vi "Actor Core.vi"(8 "error in":errorcluster, 11 "LabActor in":refnum<class "LabActor.lvclass">) -> (0 "error out":errorcluster, 3 "Actor out":refnum<class "Actor.lvclass">)   [LabVIEW 2020, in "LabActor.lvclass"]
doc: "(<B>Filename</B>: Actor Framework.lvlib:Actor.lvclass:Actor Core.vi)\n\nReceives messages to the actor, reacts to them, and initiates any error handling that may shut the actor down.\n\nDescendant classes may override this VI to append parallel tasks for the actor to complete while it handles messages. Overrides use the Call Parent Method node."
uses:
  LabActor.lvclass
  C:/GitHub/LabActor/Controllers/Application Controller/Application Controller.lvclass
  C:/GitHub/LabActor/Template Module/Template Module.lvclass
  C:/Program Files/National Instruments/LabVIEW 2020/vi.lib/ActorFramework/Actor/Actor.lvclass
  <vilib>/ActorFramework/Actor/Actor.lvclass
  NHMFL_Core/Libraries/Queued Listbox/Queued Listbox.xctl
  <vilib>/Utility/miscctls.llb/LVRectTypeDef.ctl
  <vilib>/Utility/miscctls.llb/LVPointTypeDef.ctl
  LabActor.lvclass/LabActor.ctl
  Controllers/Application Controller/Application Controller.lvclass/Application Controller.ctl
  Template Module/Template Module.lvclass/Template Module.ctl
  <vilib>/ActorFramework/Actor/Actor.lvclass/Actor.ctl
  <vilib>/ActorFramework/Message Enqueuer/Message Enqueuer.lvclass/Message Enqueuer.ctl
  Controllers/Application Controller Messages/Pulse Acquired Result/Pulse Acquired Result.lvclass
  C:/GitHub/LabActor/Template Module Messages/Result Reply Msg/Result Reply Msg.lvclass
  Controllers/Application Controller Messages/Pulse Acquired Result/Pulse Acquired Result.lvclass/Pulse Acquired Result.ctl
  LabActor Messages/Start Pulse Measurements Msg/Start Measurements Command Msg.lvclass/Start Measurements Command Msg.ctl
  LabActor Messages/Stop Measurements Command Msg/Stop Measurements Command Msg.lvclass/Stop Measurements Command Msg.ctl
  Worker Messages/Pause Work Msg/Pause Work Msg.lvclass
  C:/Program Files/National Instruments/LabVIEW 2020/vi.lib/ActorFramework/Message/Message.lvclass
  Worker Messages/Un-Pause Work Msg/Un-Pause Work Msg.lvclass
  Template Module Messages/Message Nested Object Msg/Message Nested Object Msg.lvclass/Message Nested Object Msg.ctl
  Template Module Messages/Open Item Msg/Open Item Msg.lvclass/Open Item Msg.ctl
  Template Module Messages/Save Configuration Msg/Save Configuration Msg.lvclass/Save Configuration Msg.ctl
  Plots/Plot types.ctl
  Controllers/Application Controller Messages/Open Waveform File Plot Msg/Open Waveform File Plot Msg.lvclass/Open Waveform File Plot Msg.ctl
  Controllers/Application Controller Messages/Pulse Acquired Result/Write Open plot.vi
  Controllers/Application Controller/Write Armed ref.vi
  Controllers/Application Controller/Write Devices armed.vi
  Controllers/Application Controller/Write Monitor Running.vi
  Controllers/Application Controller/Write Monitor ref.vi
  Controllers/Application Controller/Write Postproc ref.vi
  Template Module/Read stop event.vi
  Template Module/Read Open item event.vi
  Controllers/Application Controller/Read Monitor start event.vi
  Controllers/Application Controller/Read Monitor stop event.vi
  <vilib>/ActorFramework/Message Enqueuer/Init from Existing Queue.vi
  <vilib>/ActorFramework/Message Enqueuer/Enqueue.vi
  <vilib>/ActorFramework/Stop Msg/Stop Msg.lvclass
  LabActor Messages/Start Pulse Measurements Msg/Start Measurements Command Msg.lvclass
  LabActor Messages/Stop Measurements Command Msg/Stop Measurements Command Msg.lvclass
  Template Module Messages/Message Nested Object Msg/Message Nested Object Msg.lvclass
  Template Module Messages/Open Item Msg/Open Item Msg.lvclass
  Template Module Messages/Save Configuration Msg/Save Configuration Msg.lvclass
  Controllers/Application Controller Messages/Open Waveform File Plot Msg/Open Waveform File Plot Msg.lvclass
  <vilib>/ActorFramework/Message Priority Queue/Priority Enqueue.vi
  Controllers/Application Controller/Application Controller.lvclass
  <vilib>/ActorFramework/Message Enqueuer/Message Enqueuer.lvclass
  Template Module Messages/Restore Configuration Msg/Restore Configuration Msg.lvclass
  C:/GitHub/LabActor/Template Module Messages/Self-Addressed Msg/Self-addressed Msg.lvclass
  C:/GitHub/LabActor/Controllers/Application Controller Messages/Pulse Acquired Result/Pulse Acquired Result.lvclass
  C:/GitHub/LabActor/Controllers/Process Controller/Process Controller.lvclass
  C:/GitHub/LabActor/Worker/Worker.lvclass
  C:/GitHub/LabActor/LabActor/LabActor.lvclass
  C:/GitHub/LabActor/Worker Messages/Pause Work Msg/Pause Work Msg.lvclass
  C:/GitHub/LabActor/Worker Messages/Un-Pause Work Msg/Un-Pause Work Msg.lvclass
panel:
  in  "Error log":bool
  out "Origin":T1
  out "Front Panel Window:Panel Bounds":T2
  out "Devices armed":bool[](array[boolean])
  in  "About Button":bool
  in  "Pause":bool
  in  "Disarm":bool
  in  "Full XY Plot":bool
  out "Monitor file":path caption="Monintor\nFile"
  in  "View Waveform":bool
  out "PEAK FIELD":dbl format="%#.2f"
  in  "Exit":bool
  in  "Monitor configuration":bool
  in  "Pulse configuration":bool
  out "Pulse file":path caption="Pulse\nFile"
  in  "Write cfg":bool
  in  "Read cfg":bool
  in  "View XY Plot":bool
  out "Monitor Running":bool
  out "Armed":bool
  in  "Arm":bool
  in  "Stop monitor":bool
  in  "Start monitor":bool
  in  "Monitor":string[](xcontrol)
  in  "Process Pulse":string[](xcontrol)
  in  "Acquire Pulse":string[](xcontrol)
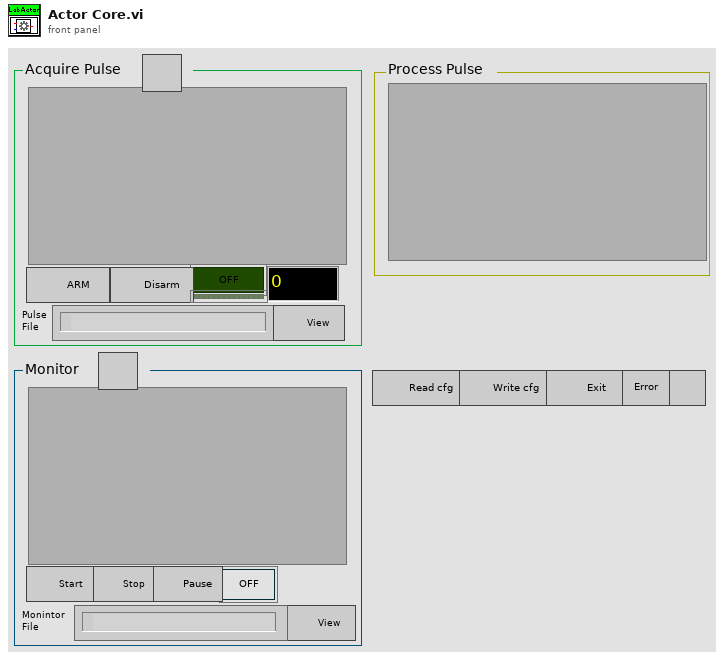
[diagram p1: front panel]
types:
  T1 = typedef "LVPointTypeDef.ctl" = cluster{"Horizontal":i16, "Vertical":i16}
  T2 = typedef "LVRectTypeDef.ctl" = cluster{"Left":i16, "Top":i16, "Right":i16, "Bottom":i16}
  T3 = typedef "Plot types.ctl" = enum16{"Waveform Plot", "XY Plot", "Full XY"}
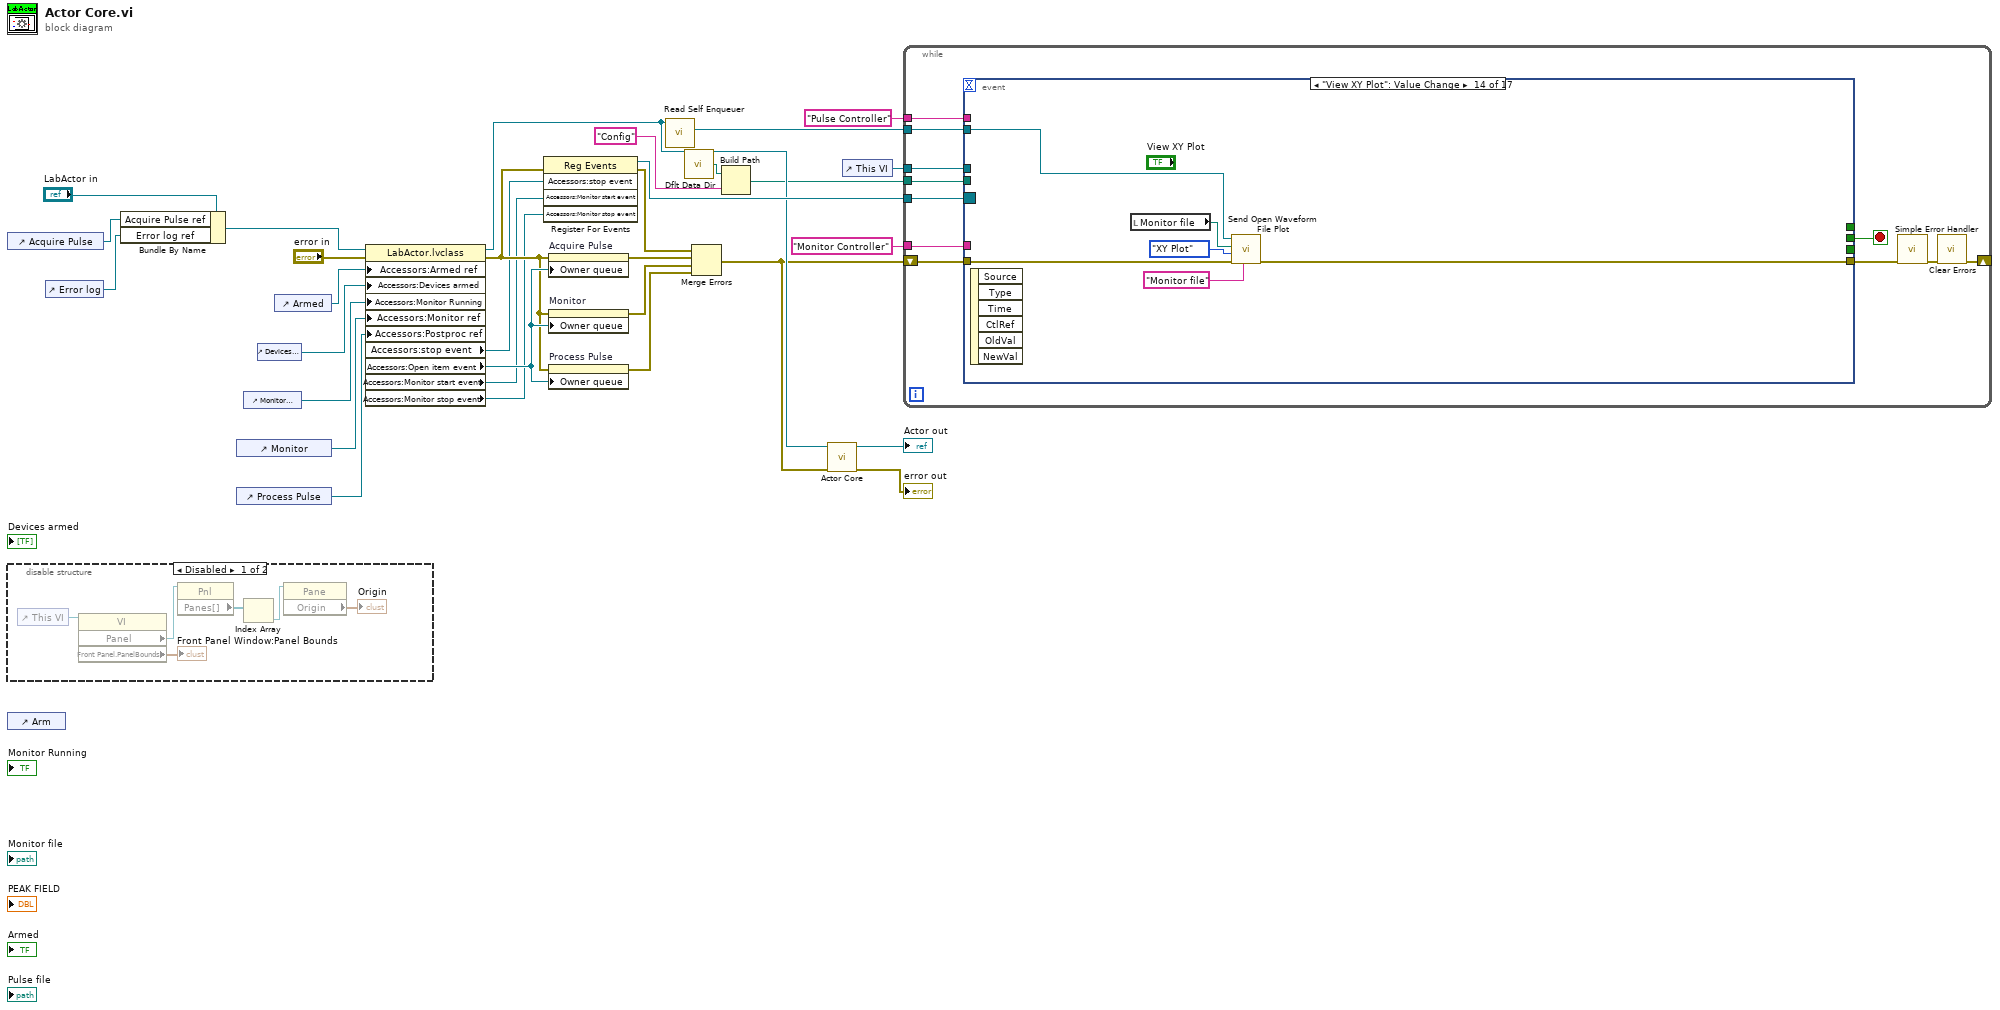
[diagram p0: block diagram]
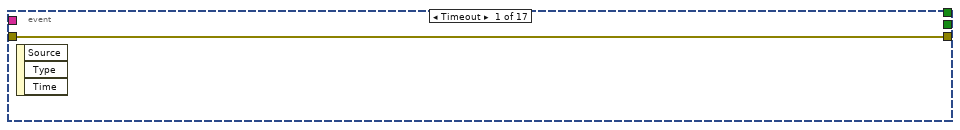
[diagram p3: hidden frame]
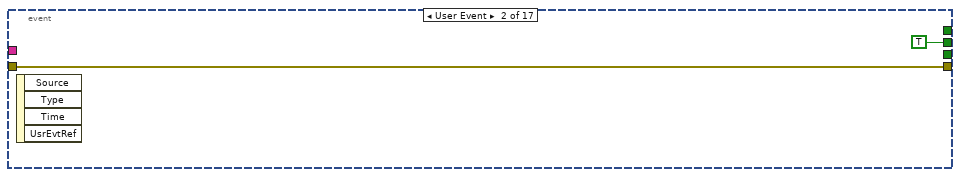
[diagram p4: hidden frame]
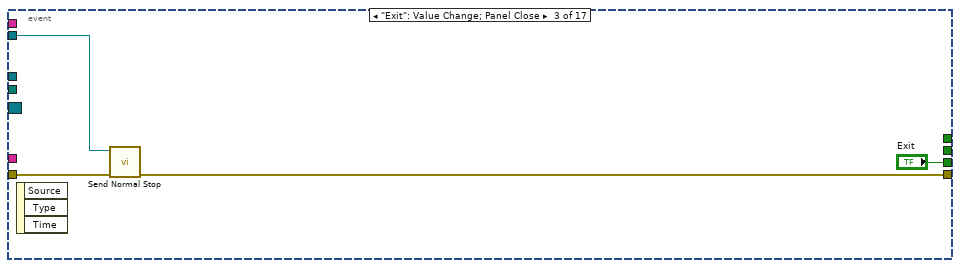
[diagram p5: hidden frame]
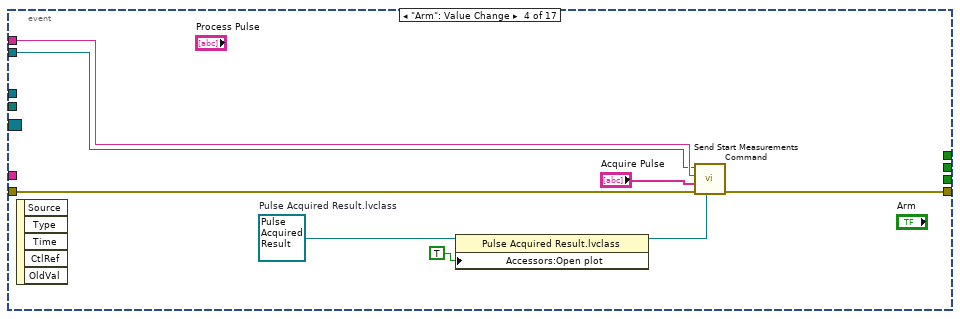
[diagram p6: hidden frame]
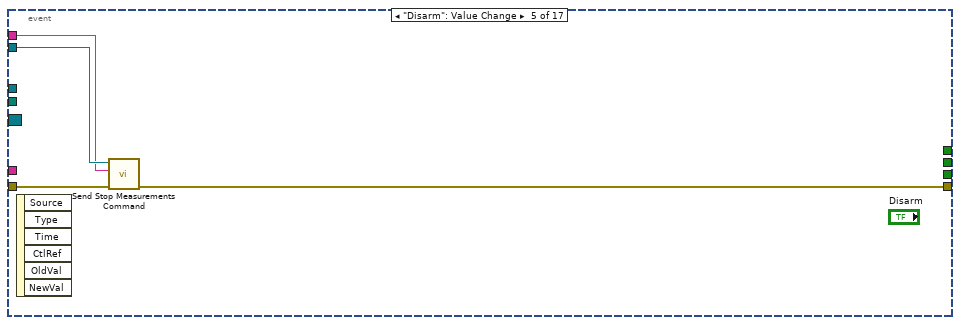
[diagram p7: hidden frame]
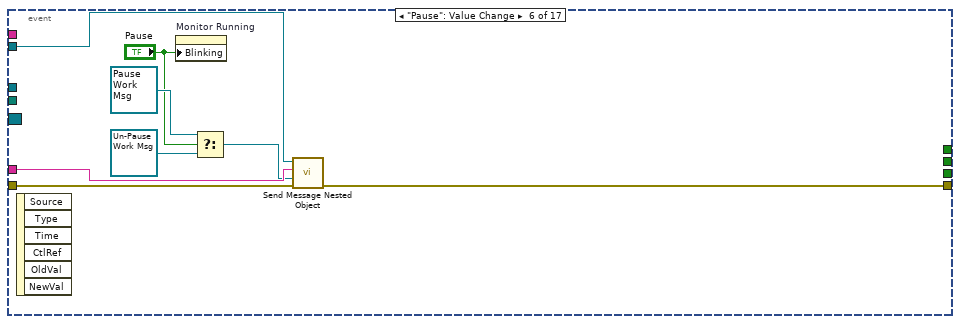
[diagram p8: hidden frame]
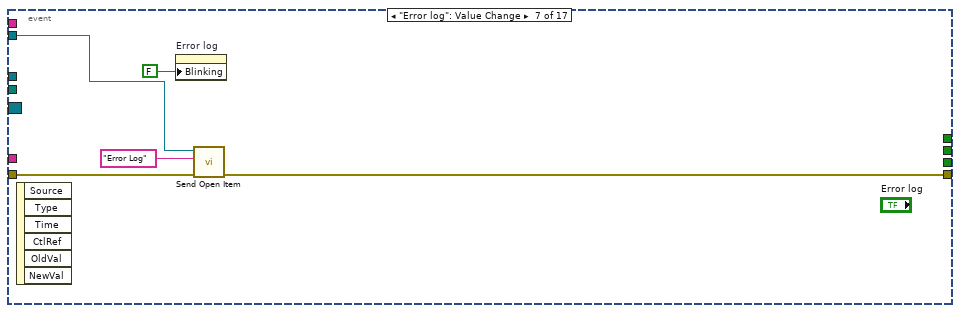
[diagram p9: hidden frame]
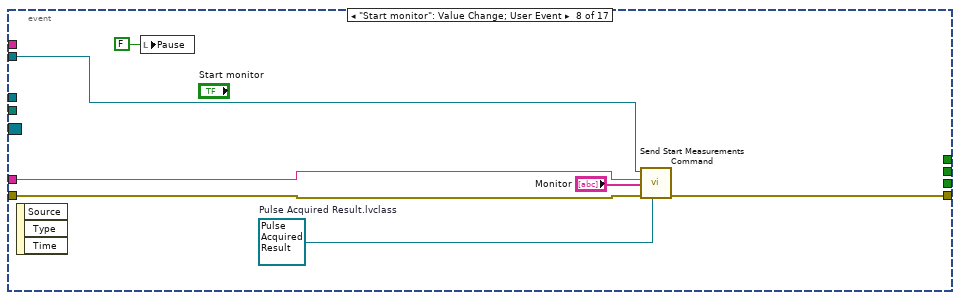
[diagram p10: hidden frame]
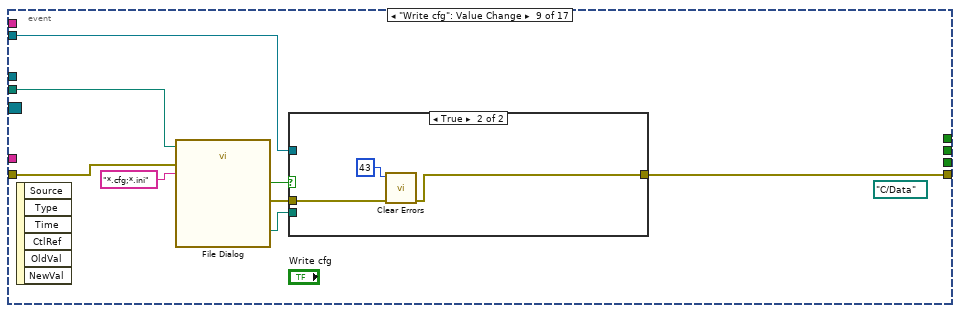
[diagram p11: hidden frame]
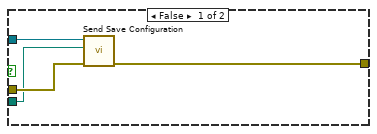
[diagram p12: hidden frame]
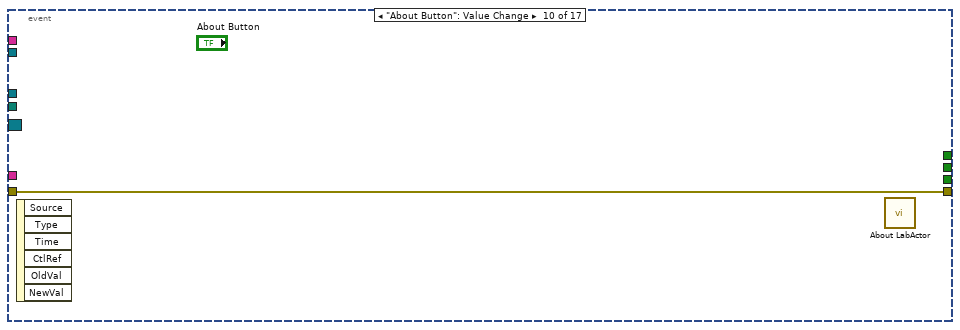
[diagram p13: hidden frame]
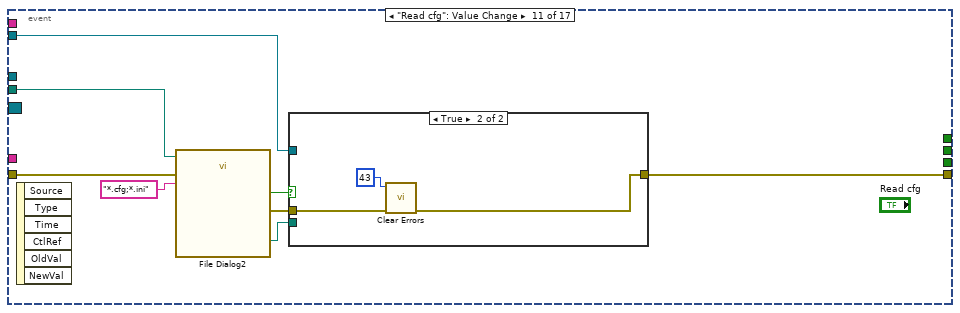
[diagram p14: hidden frame]
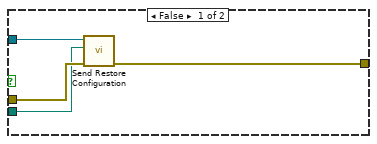
[diagram p15: hidden frame]
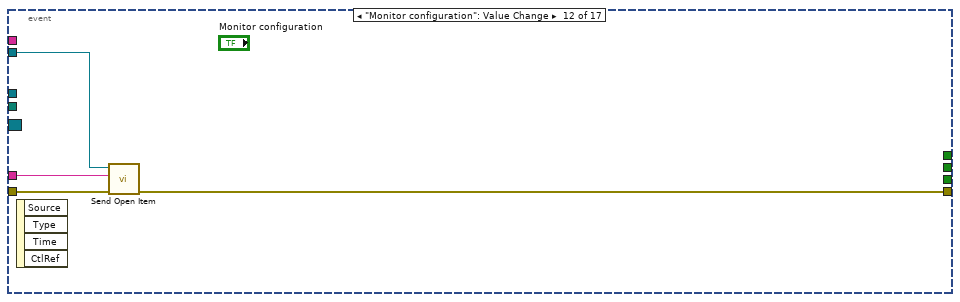
[diagram p16: hidden frame]
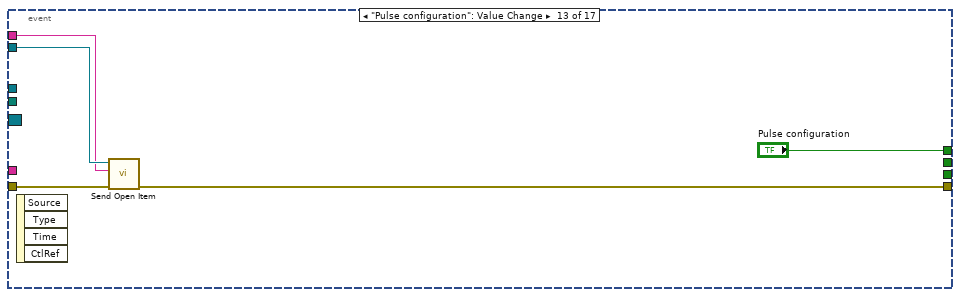
[diagram p17: hidden frame]
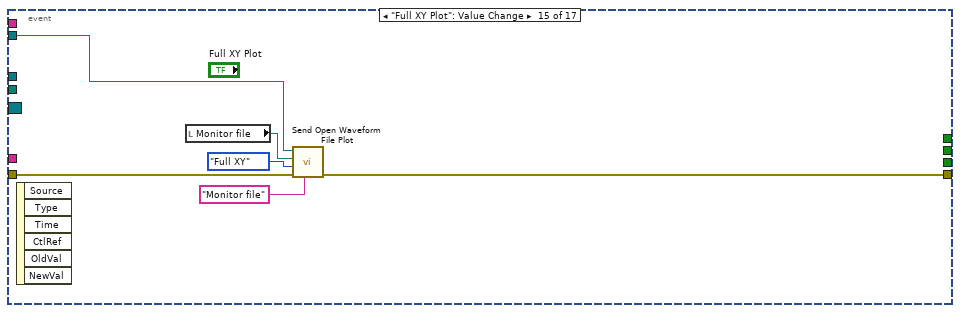
[diagram p18: hidden frame]
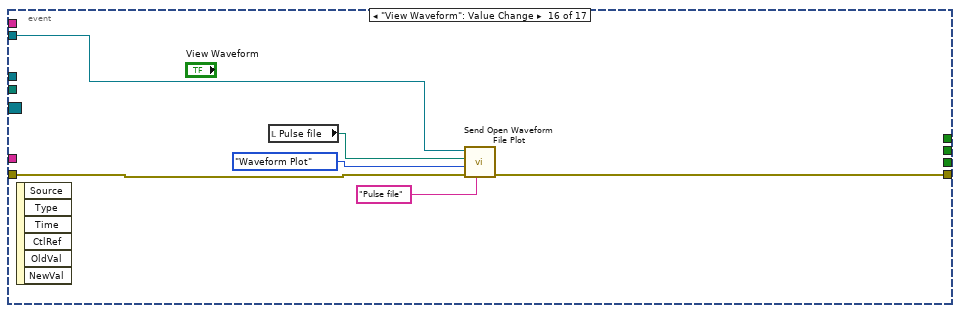
[diagram p19: hidden frame]
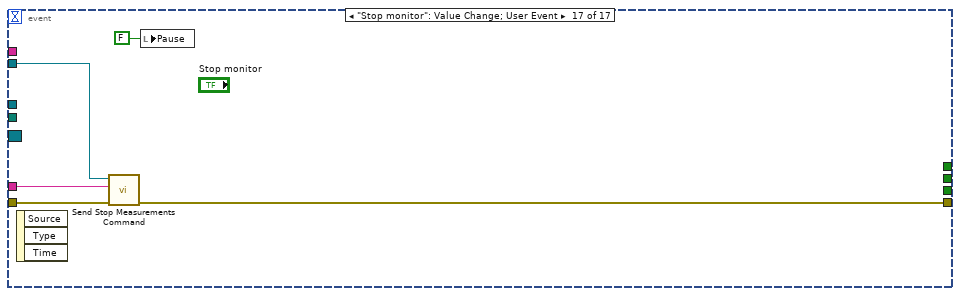
[diagram p20: hidden frame]
diagram:
  n1 = control-ref of="Acquire Pulse"() -> (w18:refnum<vi>)
  n2 = disable-structure shown="Disabled" {
    frame Disabled {
      n3 = control-ref of="This VI"() -> (w37:refnum<vi>)
      n4 = property class="VI"(reference=w37) -> ("Panel"=w35:refnum<vi>, "Front Panel.PanelBounds"=→"Front Panel Window:Panel Bounds":T2)  [unwired: 1 in, 2 out]
      n5 = property class="Pnl"(reference=w35) -> ("Panes[]"=w34:refnum<vi>[])  [unwired: 1 in, 2 out]
      n6 = Index Array(array=w34) -> (element=w33:refnum<vi>)  [unwired: 1 in]
      n7 = property class="Pane"(reference=w33) -> ("Origin"=→"Origin":T1)  [unwired: 1 in, 2 out]
    }
    frame Enabled {
    }
  }
  n8 = control-ref of="Arm"() -> ()  [unwired: 1 out]
  n9 = control-ref of="Error log"() -> (w1:refnum<vi>)
  n10 = Bundle By Name(cluster="LabActor in", "Acquire Pulse ref"=w18, "Error log ref"=w1) -> (w9:refnum<class "LabActor.lvclass">)
  n11 = control-ref of="Monitor"() -> (w12:refnum<vi>)
  n12 = control-ref of="Process Pulse"() -> (w11:refnum<vi>)
  n13 = control-ref of="Monitor Running"() -> (w13:refnum<vi>)
  n14 = control-ref of="Devices armed"() -> (w4:refnum<vi>)
  n15 = control-ref of="Armed"() -> (w14:refnum<vi>)
  n16 = property class="LabActor.lvclass"(reference=w9, error in="error in", "Accessors:Armed ref"=w14, "Accessors:Devices armed"=w4, "Accessors:Monitor Running"=w13, "Accessors:Monitor ref"=w12, "Accessors:Postproc ref"=w11) -> (reference out=w20:refnum<class "LabActor.lvclass">, error out=w23:errorcluster, "Accessors:stop event"=w15:refnum<user-event>, "Accessors:Open item event"=w27:refnum<user-event>, "Accessors:Monitor start event"=w3:refnum<user-event>, "Accessors:Monitor stop event"=w2:refnum<user-event>)
  n17 = register-events(error in=w23, w15, w3, w2) -> (reference out=w28:refnum<event-registration>, error out=w22:errorcluster)  [unwired: 1 in]
  n18 = property on="Acquire Pulse" class="Queued Listbox (strict)"(error in=w23, "Owner queue"=w27) -> (error out=w26:errorcluster)  [unwired: 1 in, 1 out]
  n19 = property on="Monitor" class="Queued Listbox (strict)"(error in=w23, "Owner queue"=w27) -> (error out=w25:errorcluster)  [unwired: 1 in, 1 out]
  n20 = property on="Process Pulse" class="Queued Listbox (strict)"(error in=w23, "Owner queue"=w27) -> (error out=w24:errorcluster)  [unwired: 1 in, 1 out]
  n21 = call <vilib>:"Read Self Enqueuer.vi"("Actor"=w20) -> ("Self Enqueuer"=w19:refnum<class "Message Enqueuer.lvclass">)  [unwired: 10 in]
  n22 = call <vilib>:"Dflt Data Dir.vi"() -> ("App:Default Data Directory"=w7:path)
  n23 = Merge Errors(w22, w26, w25, w24) -> (w10:errorcluster)
  n24 = Build Path(base path=w7, name or relative path="Config") -> (appended path=w5:path)
  n25 = call-parent "Actor Core.vi"("error in"=w10, "Measure Object in"=w20) -> ("error out"=→"error out":errorcluster, "Actor out"=→"Actor out":refnum<class "Actor.lvclass">)  [unwired: 8 in]
  n26 = control-ref of="This VI"() -> (w8:refnum<vi>)
  n27 = while {
    tunnel: w28 -> [w48]
    tunnel: w19 -> [w46]
    tunnel: "Monitor Controller" ("Controller name") -> [w45]
    tunnel: "Pulse Controller" ("Item name") -> [w44]
    shift-right: [w40] -> _
    shift-left: w10 -> [w43]
    tunnel: w8 -> [w39]
    tunnel: w5 -> [w38]
    stop <- w47 stop-if-true
    n28 = event shown="[13] \"View XY Plot\": Value Change" {
      selector: w48 -> [_ _ _ _ _ _ _ _ _ _ _ _ _ _ _ _ _]
      dyn-events: _ -> [_ _ _ _ _ _ _ _ _ _ _ _ _ _ _ _ _]
      timeout: _ -> [_ _ _ _ _ _ _ _ _ _ _ _ _ _ _ _ _]
      tunnel: [_ TRUE _ _ _ _ _ _ _ _ _ _ _ _ _ _ _] -> w47
      tunnel: w46 -> [_ _ w54 w58 w67 w71 w78 w86 w92 _ w108 w122 w126 w133 w139 w144 w150]
      tunnel: [_ _ _ _ _ _ _ _ _ _ _ _ "Pulse configuration" _ _ _ _] -> _
      tunnel: [_ _ "Exit" _ _ _ _ _ _ _ _ _ _ _ _ _ _] -> _
      tunnel: w45 -> [_ _ _ _ _ w75 _ w85 _ _ _ w121 _ _ _ _ w149]
      tunnel: w44 -> [_ _ _ w62 w66 _ _ _ _ _ _ _ w125 _ _ _ _]
      tunnel: w43 -> [w49 w50 w53 w57 w65 w69 w79 w82 w90 w103 w106 w120 w124 w129 w135 w141 w147]
      tunnel: [w49 w50 w52 w56 w64 w68 w76 w81 w89 w103 w105 w119 w123 w128 w134 w140 w146] -> w42
      tunnel: w39 -> [_ _ _ _ _ _ _ _ _ _ _ _ _ _ _ _ _]
      tunnel: w38 -> [_ _ _ _ _ _ _ _ w88 _ w104 _ _ _ _ _ _]
      event Timeout {
        n29 = event-data() -> ()  [unwired: 1 in, 3 out]
      }
      event User Event {
        n30 = event-data() -> ()  [unwired: 1 in, 4 out]
      }
      event "Exit": Value Change; Panel Close {
        n31 = event-data() -> ()  [unwired: 1 in, 3 out]
        n32 = call <vilib>:"Send Normal Stop.vi"("error in (no error)"=w53, "Message Enqueuer"=w54) -> ("error out"=w52:errorcluster)  [unwired: 9 in]
      }
      event "Arm": Value Change {
        w61 = refnum<class "Pulse Acquired Result.lvclass"> refnum  # Pulse Acquired Result.lvclass
        n33 = event-data() -> ()  [unwired: 1 in, 5 out]
        n34 = property class="Pulse Acquired Result.lvclass"(reference=w61, "Accessors:Open plot"=TRUE ("Open plot")) -> (reference out=w60:refnum<class "Pulse Acquired Result.lvclass">)  [unwired: 1 in, 1 out]
        n35 = call "Send Start Measurements Command.vi"("Reply to me"=w60, "error in (no error)"=w57, "Objects"="Acquire Pulse", "Controller name"=w62, "Message Enqueuer"=w58) -> ("error out"=w56:errorcluster)  [unwired: 5 in, 1 out]
      }
      event "Disarm": Value Change {
        n36 = event-data() -> ()  [unwired: 1 in, 6 out]
        n37 = call "Send Stop Measurements Command.vi"("error in (no error)"=w65, "Measurement Controller"=w66, "Message Enqueuer"=w67) -> ("error out"=w64:errorcluster)  [unwired: 7 in, 1 out]
      }
      event "Pause": Value Change {
        n38 = event-data() -> ()  [unwired: 1 in, 6 out]
        n39 = property on="Monitor Running" class="Bool (strict)"("Blinking"="Pause") -> ()  [unwired: 2 in, 2 out]
        n40 = Select(t=refnum<class "Pause Work Msg.lvclass"> refnum ("Pause Work Msg.lvclass"), s="Pause", f=refnum<class "Un-Pause Work Msg.lvclass"> refnum ("Un-Pause Work Msg.lvclass")) -> (s? t:f=w72:refnum<class "Message.lvclass">)
        n41 = call "Send Message Nested Object.vi"("error in (no error)"=w69, "Message"=w72, "Name"=w75, "Message Enqueuer"=w71) -> ("error out"=w68:errorcluster)  [unwired: 6 in, 1 out]
      }
      event "Error log": Value Change {
        n42 = event-data() -> ()  [unwired: 1 in, 6 out]
        n43 = property on="Error log" class="Bool"("Blinking"=FALSE) -> ()  [unwired: 2 in, 2 out]
        n44 = call "Send Open Item.vi"("error in (no error)"=w79, "Item name"="Error Log", "Message Enqueuer"=w78) -> ("error out"=w76:errorcluster)  [unwired: 7 in, 1 out]
      }
      event "Start monitor": Value Change; User Event {
        w84 = refnum<class "Pulse Acquired Result.lvclass"> refnum  # Pulse Acquired Result.lvclass
        n45 = event-data() -> ()  [unwired: 1 in, 3 out]
        n46 = local write "Pause"(FALSE ("Pause")) -> ()
        n47 = call "Send Start Measurements Command.vi"("Reply to me"=w84, "error in (no error)"=w82, "Objects"="Monitor", "Controller name"=w85, "Message Enqueuer"=w86) -> ("error out"=w81:errorcluster)  [unwired: 5 in, 1 out]
      }
      event "Write cfg": Value Change {
        (unwired) path "C:/Data" ("start path")
        n48 = event-data() -> ()  [unwired: 1 in, 6 out]
        n49 = call "File Dialog"("start path"=w88, "error in"=w90, "pattern (all files)"="*.cfg;*.ini") -> ("selected path"=w94:path, "cancelled"=w95:bool, "error out"=w91:errorcluster)  [unwired: 9 in, 1 out]
        n50 = case shown="True" w95 {
          tunnel: w94 -> [w97 _]
          tunnel: w92 -> [w99 _]
          tunnel: w91 -> [w98 w102]
          tunnel: [w96 w101] -> w89
          frame False {
            n51 = call "Send Save Configuration.vi"("error in (no error)"=w98, "File path"=w97, "Message Enqueuer"=w99) -> ("error out"=w96:errorcluster)  [unwired: 7 in, 1 out]
          }
          frame True {
            n52 = call <vilib>:"Clear Errors.vi"("error in (no error)"=w102, "specific error code to clear (0: all)"=43) -> ("error out"=w101:errorcluster)  [unwired: 4 in, 1 out]
          }
        }
      }
      event "About Button": Value Change {
        n53 = event-data() -> ()  [unwired: 1 in, 6 out]
        n54 = call "About LabActor.vi"() -> ()  [unwired: 11 in, 1 out]
      }
      event "Read cfg": Value Change {
        n55 = event-data() -> ()  [unwired: 1 in, 6 out]
        n56 = call "File Dialog2"("start path"=w104, "error in"=w106, "pattern (all files)"="*.cfg;*.ini") -> ("selected path"=w111:path, "cancelled"=w107:bool, "error out"=w109:errorcluster)  [unwired: 9 in, 1 out]
        n57 = case shown="True" w107 {
          tunnel: w111 -> [w113 _]
          tunnel: w108 -> [w115 _]
          tunnel: w109 -> [w114 w118]
          tunnel: [w112 w117] -> w105
          frame False {
            n58 = call "Send Restore Configuration.vi"("error in (no error)"=w114, "File path"=w113, "Message Enqueuer"=w115) -> ("error out"=w112:errorcluster)  [unwired: 7 in, 1 out]
          }
          frame True {
            n59 = call <vilib>:"Clear Errors.vi"("error in (no error)"=w118, "specific error code to clear (0: all)"=43) -> ("error out"=w117:errorcluster)  [unwired: 4 in, 1 out]
          }
        }
      }
      event "Monitor configuration": Value Change {
        n60 = event-data() -> ()  [unwired: 1 in, 4 out]
        n61 = call "Send Open Item.vi"("error in (no error)"=w120, "Item name"=w121, "Message Enqueuer"=w122) -> ("error out"=w119:errorcluster)  [unwired: 7 in, 1 out]
      }
      event "Pulse configuration": Value Change {
        n62 = event-data() -> ()  [unwired: 1 in, 4 out]
        n63 = call "Send Open Item.vi"("error in (no error)"=w124, "Item name"=w125, "Message Enqueuer"=w126) -> ("error out"=w123:errorcluster)  [unwired: 7 in, 1 out]
      }
      event "View XY Plot": Value Change {
        n64 = event-data() -> ()  [unwired: 1 in, 6 out]
        n65 = local read "Monitor file"() -> (w132:path)
        n66 = call "Send Open Waveform File Plot.vi"("Plot group"="Monitor file" ("Control Name"), "error in (no error)"=w129, "Plot type"=Plot_types."XY Plot", "File Path Control"=w132, "Message Enqueuer"=w133) -> ("error out"=w128:errorcluster)  [unwired: 5 in, 1 out]
      }
      event "Full XY Plot": Value Change {
        n67 = event-data() -> ()  [unwired: 1 in, 6 out]
        n68 = local read "Monitor file"() -> (w138:path)
        n69 = call "Send Open Waveform File Plot.vi"("Plot group"="Monitor file" ("Control Name"), "error in (no error)"=w135, "Plot type"=Plot_types."Full XY", "File Path Control"=w138, "Message Enqueuer"=w139) -> ("error out"=w134:errorcluster)  [unwired: 5 in, 1 out]
      }
      event "View Waveform": Value Change {
        n70 = event-data() -> ()  [unwired: 1 in, 6 out]
        n71 = local read "Pulse file"() -> (w143:path)
        n72 = call "Send Open Waveform File Plot.vi"("Plot group"="Pulse file" ("Control Name"), "error in (no error)"=w141, "Plot type"=Plot_types."Waveform Plot", "File Path Control"=w143, "Message Enqueuer"=w144) -> ("error out"=w140:errorcluster)  [unwired: 5 in, 1 out]
      }
      event "Stop monitor": Value Change; User Event {
        n73 = event-data() -> ()  [unwired: 1 in, 3 out]
        n74 = call "Send Stop Measurements Command.vi"("error in (no error)"=w147, "Measurement Controller"=w149, "Message Enqueuer"=w150) -> ("error out"=w146:errorcluster)  [unwired: 7 in, 1 out]
        n75 = local write "Pause"(FALSE ("Pause")) -> ()
      }
    }
    n76 = call <vilib>:"Simple Error Handler.vi"("error in (no error)"=w42) -> ("error out"=w41:errorcluster)  [unwired: 4 in, 4 out]
    n77 = call <vilib>:"Clear Errors.vi"("error in (no error)"=w41) -> ("error out"=w40:errorcluster)  [unwired: 5 in, 1 out]
  }
